vi "generate_script.vi"(1 "Old Component List":T2, 2 "New Component List":T2) -> (0 "Component Change Script":T1(array[cluster]))   [LabVIEW 2015]
uses:
  Systems/SystemUtil/ComponentList.ctl
  ComponentType.ctl
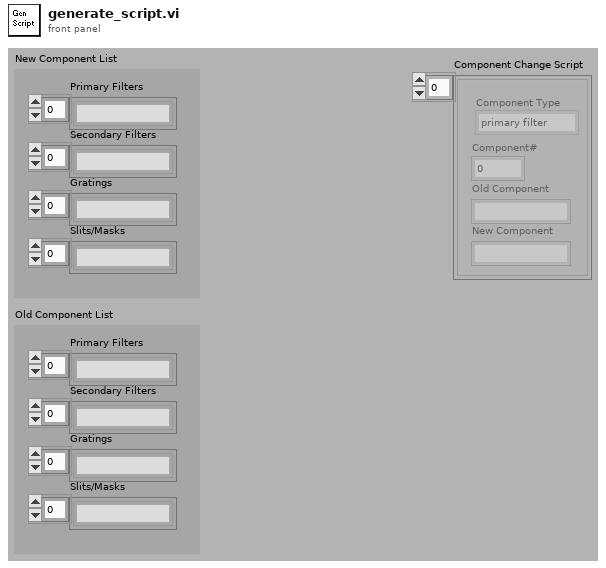
[diagram p1: front panel]
types:
  T1 = cluster{"Component Type":enum16{"primary filter", "secondary filter", "grating", "slit/mask"}, "Component#":i32, "Old Component":string, "New Component":string}[]
  T2 = typedef "ComponentList.ctl" = cluster{"Primary Filters":string[], "Secondary Filters":string[], "Gratings":string[], "Slits/Masks":string[]}
  T3 = typedef "ComponentType.ctl" = enum16{"primary filter", "secondary filter", "grating", "slit/mask"}
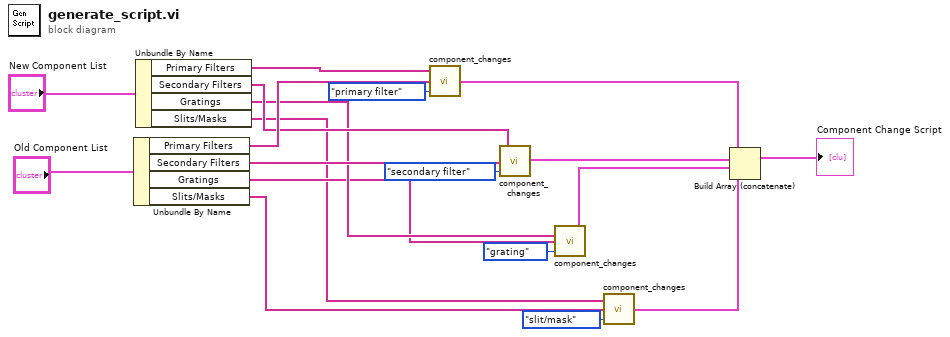
[diagram p0: block diagram]
diagram:
  n1 = Unbundle By Name("Old Component List") -> ("Primary Filters"=w16:string[], "Secondary Filters"=w14:string[], "Gratings"=w12:string[], "Slits/Masks"=w10:string[])
  n2 = Unbundle By Name("New Component List") -> ("Primary Filters"=w17:string[], "Secondary Filters"=w15:string[], "Gratings"=w13:string[], "Slits/Masks"=w11:string[])
  n3 = call "component_changes.vi"("Component Type"=ComponentType."primary filter", "Old Component List"=w16, "New Component List"=w17) -> ("Component Changes"=w9:T1)
  n4 = call "component_changes.vi"("Component Type"=ComponentType."secondary filter", "Old Component List"=w14, "New Component List"=w15) -> ("Component Changes"=w8:T1)
  n5 = call "component_changes.vi"("Component Type"=ComponentType."grating", "Old Component List"=w12, "New Component List"=w13) -> ("Component Changes"=w7:T1)
  n6 = call "component_changes.vi"("Component Type"=ComponentType."slit/mask", "Old Component List"=w10, "New Component List"=w11) -> ("Component Changes"=w6:T1)
  n7 = Build Array (concatenate)(w9, w8, w7, w6) -> (→"Component Change Script":T1)
